vi "belh.vi"(11 "Image Data":void[](array[numeric])) -> ()   [LabVIEW 2014]
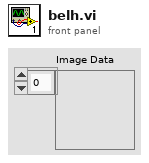
[diagram p1: front panel]
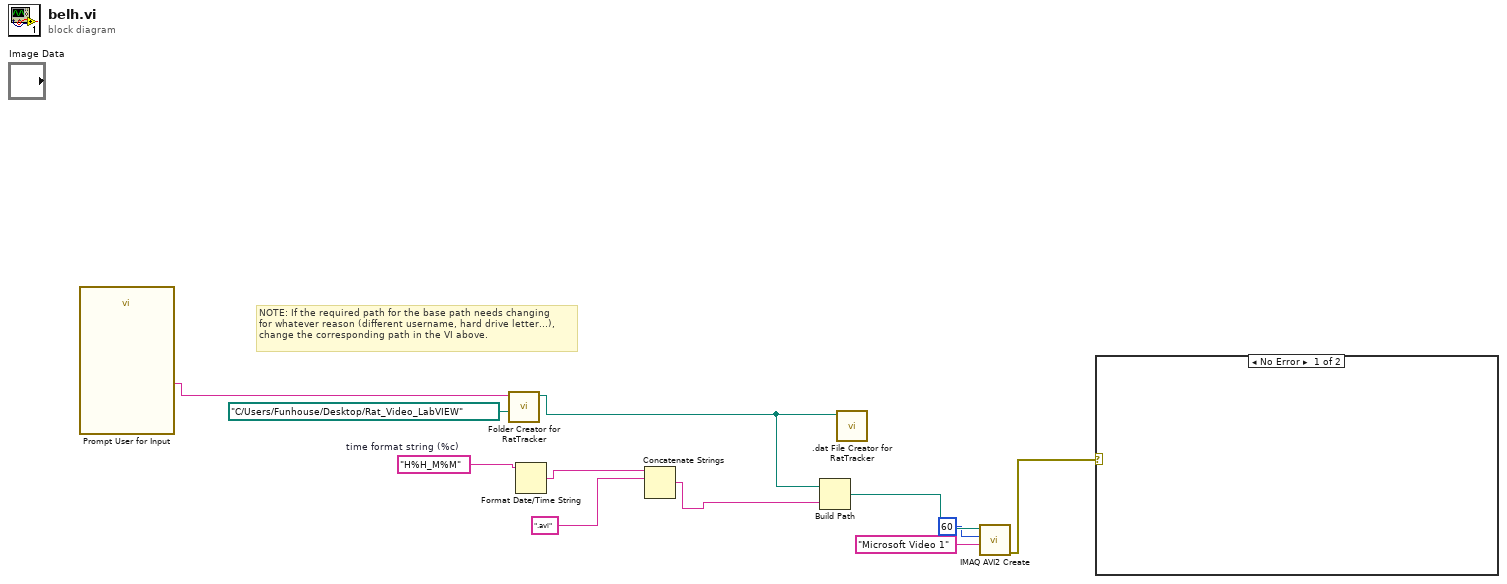
[diagram p0: block diagram]
diagram:
  w8 = "H%H_M%M"  # time format string (%c)
  # "NOTE: If the required path for the base path needs changing\nfor whatever reason (different username, hard drive letter...),\nchange the corresponding path in the VI above."
  n1 = call "Prompt User for Input"() -> ("Name"=w10:string)  [unwired: 17 in, 2 out]
  n2 = call "Folder Creator for RatTracker.vi"("Base Path"=path "C:/Users/Funhouse/Desktop/Rat_Video_LabVIEW" ("Base Path for File"), "Rat Name"=w10) -> ("Path of Folder with .avi and .dat"=w5:path)  [unwired: 9 in]
  n3 = Format Date/Time String(time format string (%c)=w8) -> (date/time string=w9:string)  [unwired: 2 in]
  n4 = Concatenate Strings(w9, ".avi") -> (w6:string)  [unwired: 2 in]
  n5 = Build Path(base path=w5, name or relative path=w6) -> (appended path=w4:path)
  n6 = call ".dat File Creator for RatTracker.vi"("Path of Folder with .avi and .dat"=w5) -> ()  [unwired: 10 in, 1 out]
  n7 = call "IMAQ AVI2 Create"("Codec"="Microsoft Video 1", "Frames Per Second"=u32 60, "AVI Path"=w4) -> ("error out"=w1:errorcluster)  [unwired: 7 in, 1 out]
  n8 = case shown="No Error" w1 {
    frame No Error {
    }
    frame Error {
    }
  }
